vi "SSI_Gpib_Data_Read.vi"(3 "字节总数":u32, 4 "error in (no error)":errorcluster, 5 "VISA resource name":refnum<visa-resource-name>) -> (0 "buffer output":string, 1 "error out":errorcluster, 2 "VISA resource ouput":refnum<visa-resource-name>)   [LabVIEW 2011]
panel:
  out "数值":i32
  in  "input buffer":string
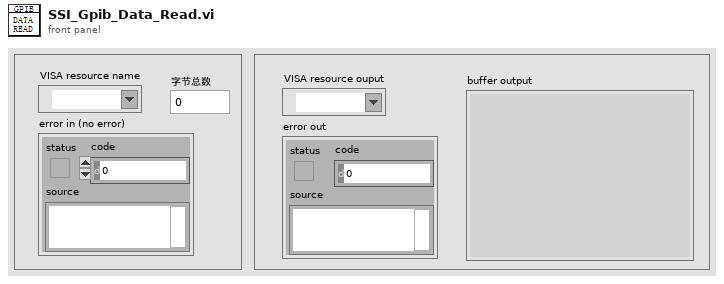
[diagram p1: front panel]
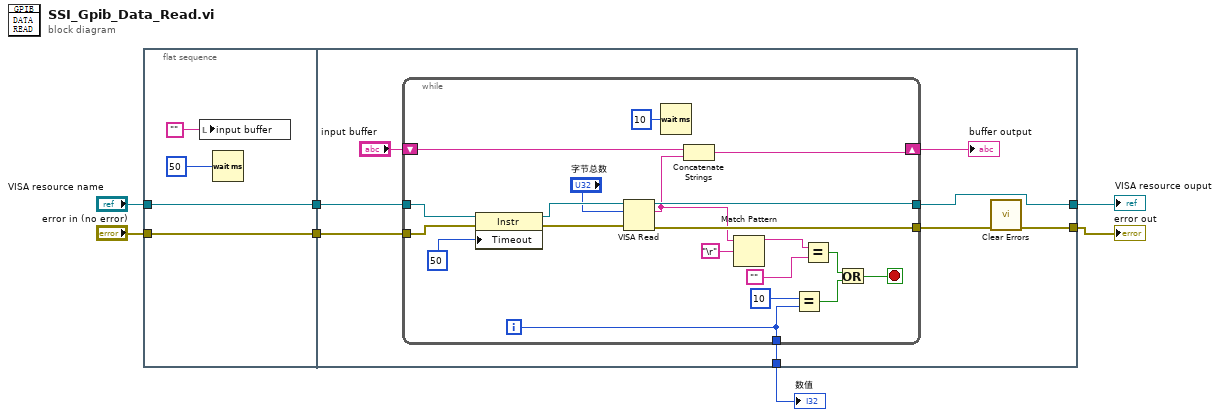
[diagram p0: block diagram]
diagram:
  n1 = flat-sequence {
    tunnel: [w9] -> w7
    tunnel: "VISA resource name" -> [w9]
    tunnel: [w8] -> w5
    tunnel: "error in (no error)" -> [w8]
    tunnel: w7 -> [w19]
    tunnel: w5 -> [w18]
    tunnel: [w16] -> w3
    tunnel: [w12] -> w2
    tunnel: [w13] -> w1
    frame #0 {
      n2 = local write "input buffer"("") -> ()
      n3 = Wait (ms)(milliseconds to wait=50) -> ()  [unwired: 1 out]
    }
    frame #1 {
      n4 = while {
        shift-right: [w36] -> w15
        shift-left: "input buffer" -> [w37]
        tunnel: [w29] -> w16
        tunnel: w19 -> [w28]
        tunnel: [w39] -> w12
        tunnel: w18 -> [w27]
        tunnel: [w38] -> w14
        i -> [w29]
        stop <- w30 stop-if-true
        n5 = property class="Instr"(reference=w28, error in=w27, "Timeout"=u32 50 ("byte count")) -> (reference out=w26:refnum<visa-resource-name>, error out=w25:errorcluster)
        n6 = VISA Read(VISA resource name=w26, byte count="字节总数", error in (no error)=w25) -> (VISA resource name out=w39:refnum<visa-resource-name>, read buffer=w21:string, error out=w38:errorcluster)  [unwired: 1 out]
        n7 = Wait (ms)(milliseconds to wait=u32 10 ("等待时间（毫秒）")) -> ()  [unwired: 1 out]
        n8 = Concatenate Strings(w37, w21) -> (w36:string)
        n9 = Match Pattern(string=w21, regular expression="\r") -> (before substring=w22:string)  [unwired: 1 in, 3 out]
        n10 = Equal?(x=10, y=w29) -> (x = y?=w32:bool)
        n11 = Equal?(x=w22, y="") -> (x = y?=w31:bool)
        n12 = Or(x=w31, y=w32) -> (x .or. y?=w30:bool)
      }
      "buffer output" <- w15
      n13 = call <vilib>:"Clear Errors.vi"("error in (no error)"=w14) -> ("error out"=w13:errorcluster)  [unwired: 6 in]
    }
  }
  "VISA resource ouput" <- w2
  "error out" <- w1
  "数值" <- w3
